vi "APU + 1 Directional Sim + 1 Dig Pattern.vi"() -> ()   [LabVIEW 2015]
uses:
  IP Source/Version Token.ctl
  IP Source/APU/Settings.ctl
  IP Source/APU/Input.ctl
  IP Source/APU/Output.ctl
  IP Source/Directional Speed/Load Input.ctl
  IP Source/Directional Speed/Input.ctl
  IP Source/Directional Speed/Settings.ctl
  IP Source/Digital Pattern Generation/Load Input.ctl
  IP Source/Digital Pattern Generation/Settings.ctl
  IP Source/Digital Pattern Generation/Input.ctl
  IP Source/APU/Shared Settings.ctl
  <vilib>/Platform/TimedLoop/XDataNode/timing_clust.ctl
  <vilib>/Platform/TimedLoop/XDataNode/nitl_modes.ctl
  <vilib>/Platform/TimedLoop/XDataNode/wakeup.ctl
  <vilib>/rvi/DataTransferAndStorage/Container/Common/niFpgaContainerGetUniqueNameForEmu.vi
  <vilib>/rvi/DataTransferAndStorage/Container/Common/niFpgaContainerSetEmuInfo.vi
  <vilib>/rvi/eio/common/nirviEmuReportErrorAndStop.vi
  <vilib>/rvi/Emulation/niFpgaSctlEmulationGetInTimedLoop.vi
  <vilib>/rvi/Emulation/niFpgaEmulationReportErrorSimple.vi
  <vilib>/rvi/Emulation/niFpgaGetClockAttributes.vi
  <vilib>/rvi/Emulation/niFpgaCriticalErrorInLSC.vi
  <vilib>/rvi/eio/common/nirviEmuTemplateMethod_errors.vi
  <vilib>/rvi/LocalResourceManager/LocalResourceManager.xnode
  <vilib>/Platform/TimedLoop/XDataNode/XDataNode.xnode
  <vilib>/eio/EIONode/EIONode.xnode
  <vilib>/Platform/TimedLoop/XDataNode/XDNodeRunTimeDep.lvlib
  IP Source/APU/APU.lvlib
  IP Source/Directional Speed/Directional Speed.lvlib
  IP Source/Digital Pattern Generation/Digital Pattern Generation.lvlib
  IP Source/Engine Simulation Toolkit.lvlib
panel:
  in  "shared settings.my apu":T1 {"start" format="%#.15g"}
  in  "go.my apu":bool
  in  "input.Pattern 1":T2
  in  "settings.Pattern 1":T3
  in  "load input.Pattern 1":T4
  in  "settings.DirectionSim":T5
  in  "input.DirectionSim":T6
  in  "load input.DirectionSim":T7
  out "output.my apu":T8 caption="output"
  in  "input.my apu":T9={"desired speed"=0.0, "reset"=TRUE} caption="input"
  in  "settings.my apu":T10 caption="settings"
  in  "est.version":T11
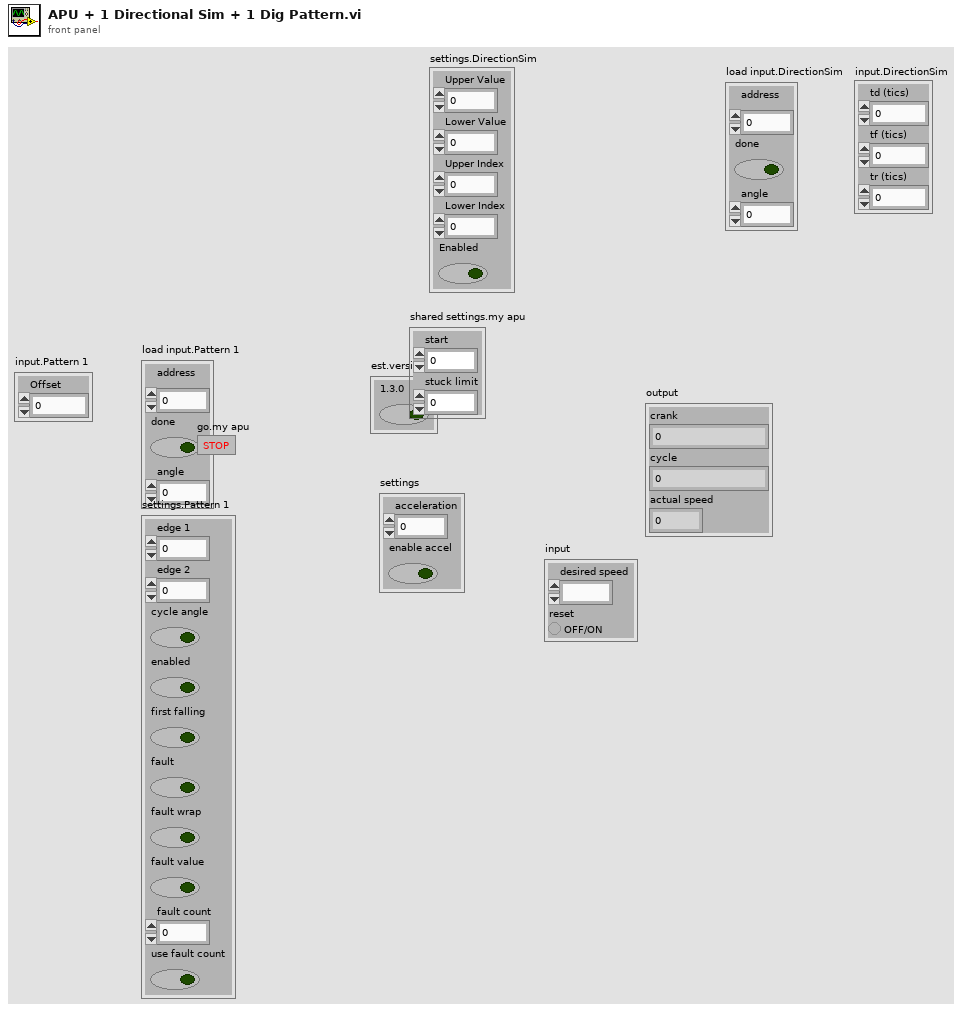
[diagram p1: front panel]
types:
  T1 = typedef "Engine Simulation Toolkit.lvlib/APU.lvlib/Shared Settings.ctl" = cluster{"start":fxp<+,17,17>, "stuck limit":fxp<+,18,18>}
  T2 = typedef "Engine Simulation Toolkit.lvlib/Digital Pattern Generation.lvlib/Input.ctl" = cluster{"Offset":i16}
  T3 = typedef "Engine Simulation Toolkit.lvlib/Digital Pattern Generation.lvlib/Settings.ctl" = cluster{"edge 1":u16, "edge 2":u16, "cycle angle":bool, "enabled":bool, "first falling":bool, "fault":bool, "fault wrap":bool, "fault value":bool, "fault count":fxp<+,4,4>, "use fault count":bool}
  T4 = typedef "Engine Simulation Toolkit.lvlib/Digital Pattern Generation.lvlib/Load Input.ctl" = cluster{"address":fxp<+,11,11>, "done":bool, "angle":u16}
  T5 = typedef "Engine Simulation Toolkit.lvlib/Directional Speed.lvlib/Settings.ctl" = cluster{"Upper Value":u16, "Lower Value":u16, "Upper Index":fxp<+,10,10>, "Lower Index":fxp<+,10,10>, "Enabled":bool}
  T6 = typedef "Engine Simulation Toolkit.lvlib/Directional Speed.lvlib/Input.ctl" = cluster{"td (tics)":u16, "tf (tics)":u16, "tr (tics)":u16}
  T7 = typedef "Engine Simulation Toolkit.lvlib/Directional Speed.lvlib/Load Input.ctl" = cluster{"address":fxp<+,10,10>, "done":bool, "angle":u16}
  T8 = typedef "Engine Simulation Toolkit.lvlib/APU.lvlib/Output.ctl" = cluster{"crank":u16, "cycle":u16, "actual speed":fxp<+/-,23,2>}
  T9 = typedef "Engine Simulation Toolkit.lvlib/APU.lvlib/Input.ctl" = cluster{"desired speed":fxp<+/-,23,2>, "reset":bool}
  T10 = typedef "Engine Simulation Toolkit.lvlib/APU.lvlib/Settings.ctl" = cluster{"acceleration":fxp<+,18,-20>, "enable accel":bool}
  T11 = typedef "Engine Simulation Toolkit.lvlib/Version Token.ctl" = cluster{"1.3.0":bool}
  T12 = typedef "XDNodeRunTimeDep.lvlib/timing_clust.ctl" = cluster{"Expected End [f-1]":u64, "Actual End [f-1]":u64, "Finished Late? [f-1]":bool, "Expected End [i-1]":u64, "Actual End [i-1]":u64, "Finished Late? [i-1]":bool, "Expected Start [i]":u64, "Actual Start [i]":u64, "Expected Start [f]":u64, "Actual Start [f]":u64, "Source Name":string, "Structure Name":string, "Period":i64, "Deadline":i64, "Offset":i64, "Start":i64, "Priority":i32, "Timeout":i32, "Mode":T13, "Wakeup Reason":T14, "Error":errorcluster, "Source Type":string, "Secondary Source Type":string, "Global End Time":u64, "Global Start Time":u64, "Frame Duration":u64, "Iteration Duration":u64, "Assigned CPU":i32, "I/O Scan Engine Mode":u32}
  T13 = typedef "XDNodeRunTimeDep.lvlib/nitl_modes.ctl" = enum32{"No Change", "Process missed periods, maintain original phase", "Discard missed periods, maintain original phase", "Process missed periods, ignore original phase", "Discard missed periods, ignore original phase"}
  T14 = typedef "XDNodeRunTimeDep.lvlib/wakeup.ctl" = enum32{"Normal", "Aborted", "Asynchronous wakeup", "Timing source error", "Timed loop error", "Timeout"}
  T15 = typedef "Engine Simulation Toolkit.lvlib/APU.lvlib/Register Bus.ctl" = cluster{"Speed":refnum<k21>, "Crank Angle":refnum<k21>, "Cycle Angle":refnum<k21>, "Crank Count":refnum<k21>, "Cycle Count":refnum<k21>, "1.25 MHz Counter":refnum<k21>, "Crank Rollover":refnum<k21>, "Cycle Rollover":refnum<k21>, "shared settings":T1}
  T16 = typedef "Engine Simulation Toolkit.lvlib/Digital Pattern Generation.lvlib/Load Data.ctl" = cluster{"max address":fxp<+,11,11>, "memory":refnum<k21>}
  T17 = typedef "Engine Simulation Toolkit.lvlib/Directional Speed.lvlib/Load Data.ctl" = cluster{"max address":fxp<+,10,10>, "Memory":refnum<k21>}
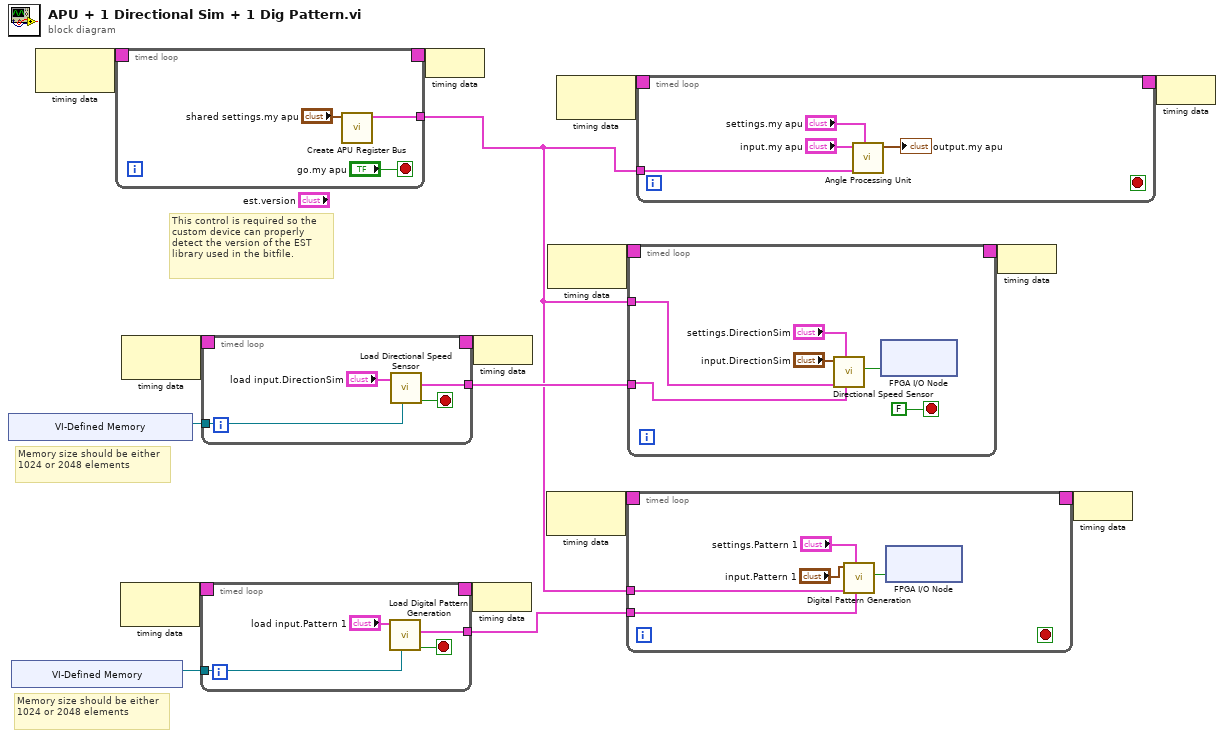
[diagram p0: block diagram]
diagram:
  # "Memory size should be either 1024 or 2048 elements"
  # "This control is required so the custom device can properly detect the version of the EST library used in the bitfile."
  # "Memory size should be either 1024 or 2048 elements"
  n1 = xnode "VI-Defined Memory"() -> ("Memory Out"=w15:refnum<k21>)
  n2 = xnode "VI-Defined Memory"() -> ("Memory Out"=w6:refnum<k21>)
  n3 = node-c288() -> (w3:T12)  [unwired: 1 in]
  n4 = timed-loop {
    timing: w3 -> [_]
    timing-out: [_] -> w2
    tunnel: [w20] -> w1
    stop <- "go.my apu" stop-if-true
    n5 = call "Create APU Register Bus.vi"("shared settings.<user name>"="shared settings.my apu") -> ("register bus"=w20:T15)  [unwired: 10 in]
  }
  n6 = node-c288() -> (w10:T12)  [unwired: 1 in]
  n7 = node-c288() -> (w17:T12)  [unwired: 1 in]
  n8 = timed-loop {
    timing: w10 -> [_]
    timing-out: [_] -> w9
    tunnel: w6 -> [w25]
    tunnel: [w24] -> w5
    stop <- w26 stop-if-true
    n9 = call "Load Digital Pattern Generation.vi"("memory"=w25, "load input.<user name>"="load input.Pattern 1") -> ("done"=w26:bool, "load data"=w24:T16)  [unwired: 8 in]
  }
  n10 = timed-loop {
    timing: w17 -> [_]
    timing-out: [_] -> w16
    tunnel: w15 -> [w31]
    tunnel: [w30] -> w4
    stop <- w32 stop-if-true
    n11 = call "Load Directional Speed Sensor.vi"("Memory In"=w31, "load input.<user name>"="load input.DirectionSim") -> ("done"=w32:bool, "load data"=w30:T17)  [unwired: 8 in]
  }
  n12 = node-c288(w2) -> ()
  n13 = node-c288(w9) -> ()
  n14 = node-c288(w16) -> ()
  n15 = node-c288() -> (w8:T12)  [unwired: 1 in]
  n16 = node-c288() -> (w14:T12)  [unwired: 1 in]
  n17 = node-c288() -> (w12:T12)  [unwired: 1 in]
  n18 = timed-loop {
    timing: w8 -> [_]
    timing-out: [_] -> w7
    tunnel: w5 -> [w36]
    tunnel: w1 -> [w35]
    stop <- _ stop-if-true
    n19 = call "Digital Pattern Generation.vi"("load data"=w36, "settings.<user name>"="settings.Pattern 1", "register bus"=w35, "input.<user name>"="input.Pattern 1") -> ("digial output"=w38:bool)  [unwired: 7 in]
    n20 = xnode "FPGA I/O Node"("DO1"=w38) -> ()  [unwired: 1 in, 1 out]
  }
  n21 = timed-loop {
    tunnel: w1 -> [w45]
    timing: w14 -> [_]
    timing-out: [_] -> w13
    tunnel: w4 -> [w44]
    stop <- FALSE stop-if-true
    n22 = call "Directional Speed Sensor.vi"("load data"=w44, "settings.<user name>"="settings.DirectionSim", "register bus"=w45, "input.<user name>"="input.DirectionSim") -> ("digial output"=w46:bool)  [unwired: 7 in]
    n23 = xnode "FPGA I/O Node"("DO0"=w46) -> ()  [unwired: 1 in, 1 out]
  }
  n24 = timed-loop {
    timing: w12 -> [_]
    timing-out: [_] -> w11
    tunnel: w1 -> [w50]
    stop <- _ stop-if-true
    n25 = call "Angle Processing Unit.vi"("settings.<user name>"="settings.my apu", "register bus"=w50, "input.<user name>"="input.my apu") -> ("output.<user name>"=→"output.my apu":T8)  [unwired: 8 in]
  }
  n26 = node-c288(w13) -> ()
  n27 = node-c288(w7) -> ()
  n28 = node-c288(w11) -> ()
